vi "weq brawer.vi"() -> ()   [LabVIEW 2014]
panel:
  in  "정지":bool
  in  "new":bool
  in  "URL":string="http://www.lightron.co.kr/"
  in  "forword":bool
  in  "back":bool
  in  "contet":bool
  in  "WebBrowser":refnum<k7>(container)
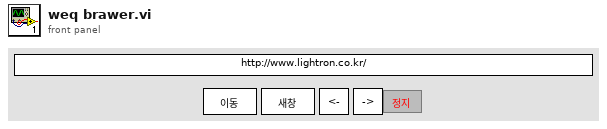
[diagram p1: front panel]
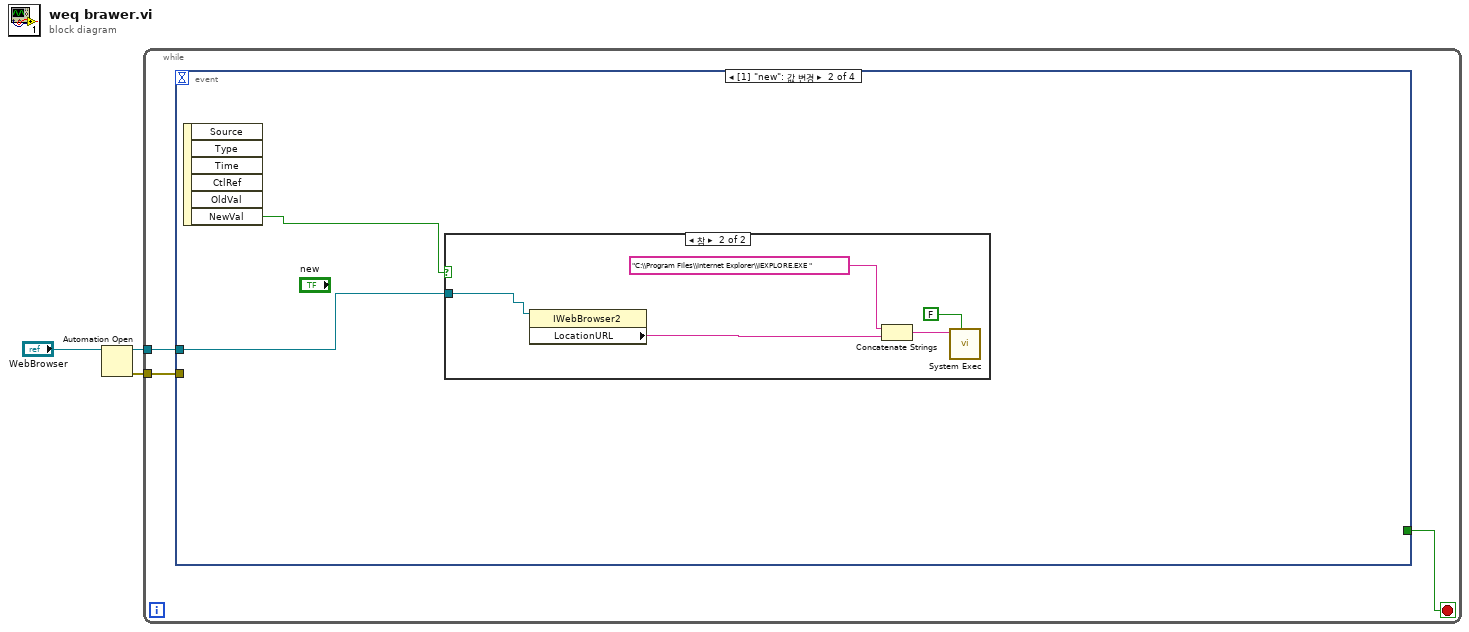
[diagram p0: block diagram]
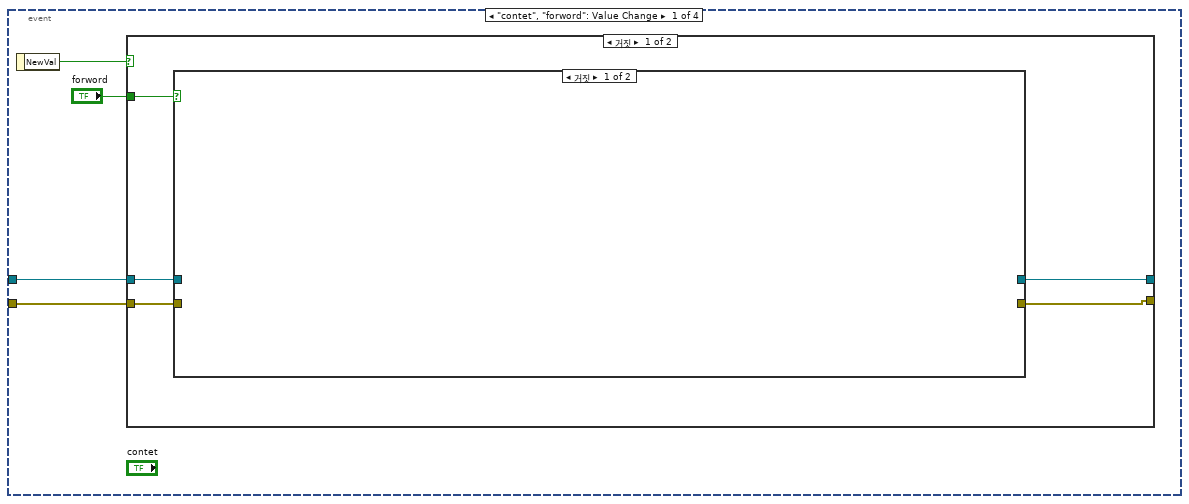
[diagram p2: hidden frame]
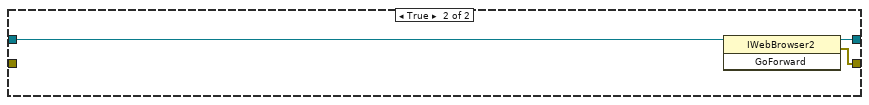
[diagram p3: hidden frame]
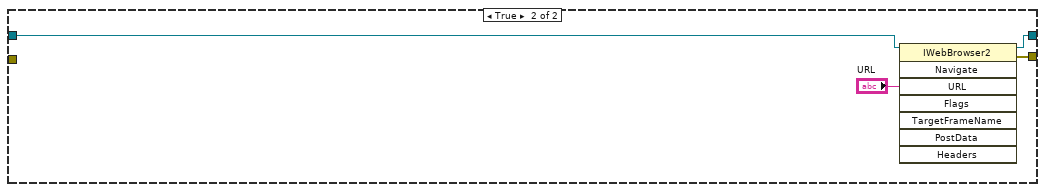
[diagram p4: hidden frame]
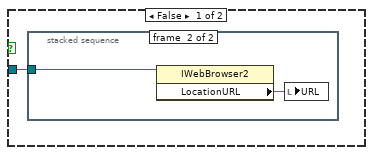
[diagram p5: hidden frame]
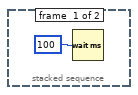
[diagram p6: hidden frame]
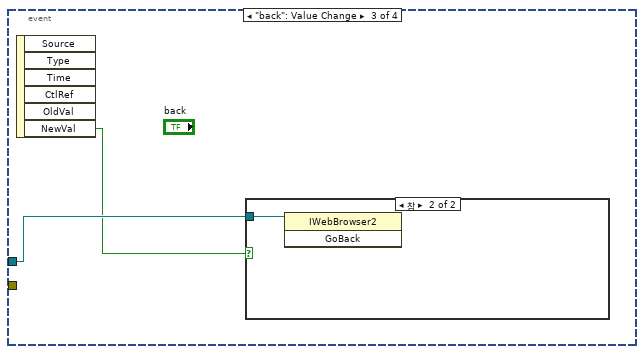
[diagram p7: hidden frame]
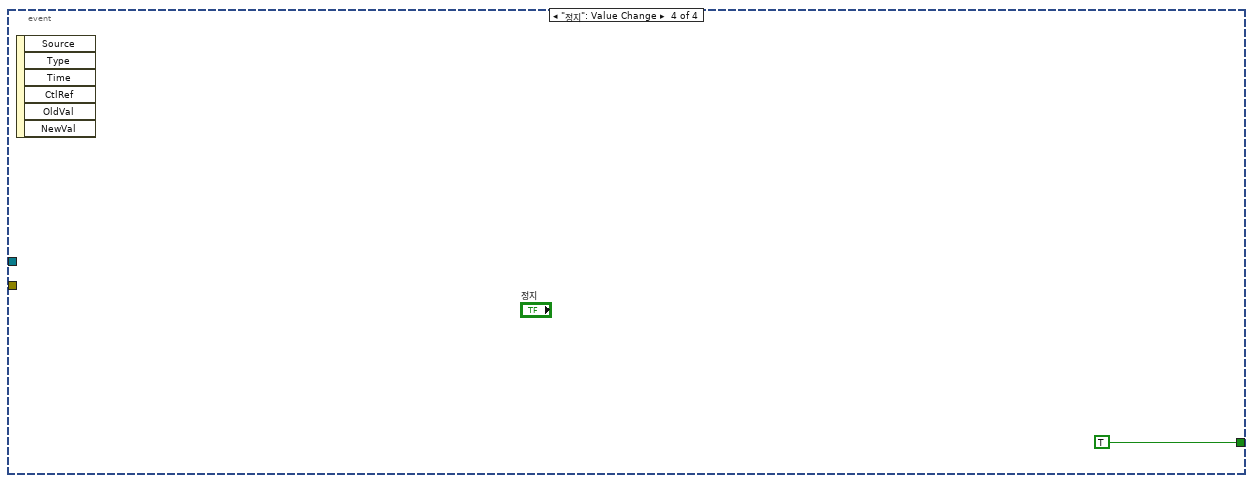
[diagram p9: hidden frame]
diagram:
  n1 = Automation Open(Automation Refnum="WebBrowser") -> (Automation Refnum=w2:refnum<k7>, error out=w1:errorcluster)  [unwired: 1 in, 2 out]
  n2 = while {
    tunnel: w2 -> [w6]
    tunnel: w1 -> [w5]
    stop <- w4 stop-if-true
    n3 = event shown="[1] \"new\": 값 변경" {
      selector: _ -> [_ _ _ _]
      dyn-events: _ -> [_ _ _ _]
      timeout: _ -> [_ _ _ _]
      tunnel: w6 -> [w10 w23 w35 _]
      tunnel: w5 -> [w7 _ _ _]
      tunnel: [_ _ _ TRUE] -> w4
      event "contet", "forword": Value Change {
        n4 = event-data() -> ("NewVal"=w9:bool)  [unwired: 1 in]
        n5 = case shown="거짓" w9 {
          tunnel: "forword" -> [w15 _]
          tunnel: [w14 w22] -> _
          tunnel: [w13 w21] -> _
          tunnel: w7 -> [w12 _]
          tunnel: w10 -> [w11 w20]
          frame False {
            n6 = case shown="거짓" w15 {
              tunnel: [_ w18] -> w14
              tunnel: [_ w17] -> w13
              tunnel: w12 -> [_ _]
              tunnel: w11 -> [_ w16]
              frame False {
              }
              frame True {
                n7 = invoke class="IWebBrowser2" method="GoForward"(reference=w16) -> (reference out=w18:refnum<k7>, error out=w17:errorcluster)  [unwired: 2 in, 1 out]
              }
            }
          }
          frame True {
            n8 = invoke class="IWebBrowser2" method="Navigate"(reference=w20, "URL"="URL") -> (reference out=w22:refnum<k7>, error out=w21:errorcluster)  [unwired: 6 in, 6 out]
          }
        }
      }
      event "new": Value Change {
        n9 = event-data() -> ("NewVal"=w24:bool)  [unwired: 1 in, 5 out]
        n10 = case shown="참" w24 {
          tunnel: w23 -> [w25 w29]
          frame False {
            n11 = stacked-sequence {
              tunnel: w25 -> [_ w27]
              frame #0 {
                n12 = Wait (ms)(milliseconds to wait=u32 100) -> ()  [unwired: 1 out]
              }
              frame #1 {
                n13 = property class="IWebBrowser2"(reference=w27) -> ("LocationURL"=w28:string)  [unwired: 1 in, 2 out]
                n14 = local write "URL"(w28) -> ()
              }
            }
          }
          frame True {
            n15 = property class="IWebBrowser2"(reference=w29) -> ("LocationURL"=w30:string)  [unwired: 1 in, 2 out]
            n16 = Concatenate Strings("C:\\Program Files\\Internet Explorer\\IEXPLORE.EXE " ("command line"), w30) -> (w33:string)
            n17 = call <vilib>:"System Exec.vi"("wait until completion? (T)"=FALSE, "command line"=w33) -> ()  [unwired: 4 in, 6 out]
          }
        }
      }
      event "back": Value Change {
        n18 = event-data() -> ("NewVal"=w34:bool)  [unwired: 1 in, 5 out]
        n19 = case shown="참" w34 {
          tunnel: w35 -> [_ w36]
          frame False {
          }
          frame True {
            n20 = invoke class="IWebBrowser2" method="GoBack"(reference=w36) -> ()  [unwired: 2 in, 3 out]
          }
        }
      }
      event "정지": Value Change {
        n21 = event-data() -> ()  [unwired: 1 in, 6 out]
      }
    }
  }
